vi "Temperature.vi"(2 "F":dbl, 3 "C":dbl) -> (0 "F to C":dbl, 1 "C to F":dbl)   [LabVIEW 2020]
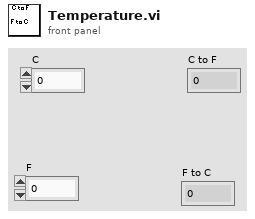
[diagram p1: front panel]
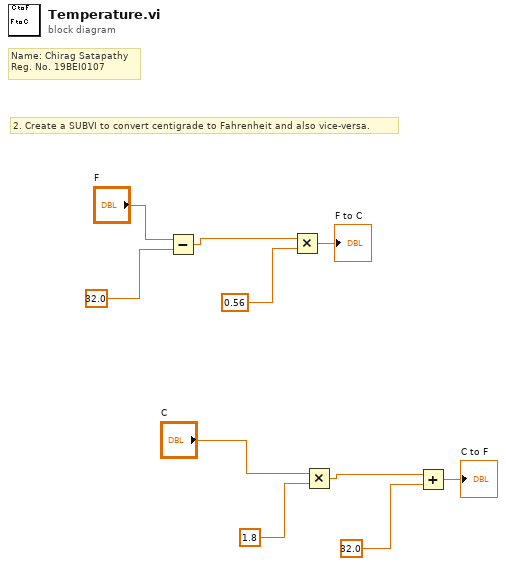
[diagram p0: block diagram]
diagram:
  # "2. Create a SUBVI to convert centigrade to Fahrenheit and also vice-versa."
  # "Name: Chirag Satapathy\nReg. No. 19BEI0107"
  n1 = Subtract(x="F", y=32.0) -> (x-y=w8:dbl)
  n2 = Multiply(x=w8, y=0.56) -> (x*y=→"F to C":dbl)
  n3 = Multiply(x="C", y=1.8) -> (x*y=w4:dbl)
  n4 = Add(x=w4, y=32.0) -> (x+y=→"C to F":dbl)
